vi "LV21_2.vi"() -> ()   [LabVIEW 2021]
panel:
  out "Numeric 3":i32
  out "Real Input 2":string="B Y\nA X\nC Z\nA Z\nB Y\nB Y\nA X\nC Z\nB Y\nB Y\nC Z\nC X\nB Y\nC Z\nB Y\nC Z\nA Z\nA Z\nA X\nB Y\nA X\nC Z\nC Y\nC Z\nC Z\nC Z\nA X\nA X\nB Y\nA Z\nB Z\nB Y\nA X\nA X\nC Z\nB Y\nB Y\nB Z\nA Z\nA X\nC Z\nB Z\nA Z\nC Z\nC Z\nC Z\nC Z\nC Z\nC Z\nB X\nA Z\nA Z\nC Z\nC Z\nC Z\nA Y\nC Z\nB Y\nC Z\nC Z\nC Z\nB Y\nB Z\nA X\nA X\nC Z\nB Y\nB Y\nB Z\nA X\nA X\nC Z\nB Y\nC Z\nA X\nC Z\nA X\nC X\nA Y\nA Y\nB Y\nA Y\nC Z\nB Y\nC Z\nC Z\nA X\nC Z\nA Z\nC Z\nA X\nC Z\nB Y\nB Y\nC Z\nB Z\nC Y\nC Z\nB Y\nC Z\nC Z\nB X\nA X\nC Z\nC Z\nB Y\nC Z\nB Y\nA Z\nB Y\nB Z\nA Z\nC Z\nC Z\nC Z\nA Z\nC Z\nA X\nA X\nA Z\nC Z\nA X\nA Z\nC Z\nA Z\nA Y\nB Y\nA Z\nB X\nA X\nC Z\nC Z\nB Y\nC Y\nB Y\nB Z\nB Y\nB Y\nC Z\nC Z\nC Z\nC Z\nA Y\nC Z\nB Z\nA X\nB Y\nA Y\nC Z\nC Z\nC Z\nC Z\nC Z\nB Y\nC Z\nB Y\nC Z\nB Y\nC Z\nC X\nA Y\nA X\nC Y\nB Y\nA Z\nC Z\nC Z\nB Y\nB Y\nA X\nB Y\nA Y\nA X\nA X\nB Y\nA X\nA X\nB Y\nC Z\nC Z\nB Y\nC Z\nA Z\nC Z\nB Z\nC Z\nA Y\nC Z\nB Z\nC Z\nA Y\nA Y\nC Z\nA X\nB Y\nC Z\nA X\nB Y\nB Y\nA X\nA X\nC Z\nB Y\nC Z\nB Z\nC Z\nA X\nC Z\nB Y\nB Y\nA X\nB Z\nC Z\nB Z\nB Y\nB Y\nA Y\nB Z\nA Z\nC Z\nC Z\nA X\nA X\nA X\nC Z\nB Y\nA X\nA Y\nC Z\nA X\nB Y\nA Y\nA Y\nC Z\nC Z\nC Z\nA Z\nB Z\nC Z\nB Y\nC Z\nC Z\nA Y\nA X\nC Z\nB Y\nC Z\nC Z\nB Y\nB Y\nA Y\nC Z\nB Y\nB Y\nA Z\nC Z\nC Z\nC Z\nC Z\nB Z\nC Z\nB Y\nA X\nC Z\nB Z\nA Z\nA X\nC Z\nA X\nA X\nB Y\nC Z\nC Z\nA X\nC Z\nA Y\nC Z\nC Z\nA X\nB Y\nC Z\nB Z\nB Y\nC Z\nA Z\nC Z\nC Z\nA Y\nA Z\nC Z\nC Z\nB Z\nC Z\nB Y\nC Z\nC Z\nA X\nC Z\nC Z\nB Z\nC Z\nB Z\nA X\nB Y\nC Z\nC Z\nC Z\nC Z\nC Z\nA Z\nA Y\nA X\nA X\nC Z\nB X\nA Z\nA X\nC Z\nB Z\nC Z\nB Y\nA Z\nC Z\nB Y\nC Z\nC Y\nA Y\nC Z\nB Y\nB Y\nC Z\nA X\nC Z\nA X\nC X\nA X\nB X\nA X\nC Z\nC Z\nC Z\nB Y\nB Y\nC Z\nB Z\nC Z\nB Y\nA X\nC X\nC Z\nB Y\nA Z\nA X\nB Y\nB Y\nC Z\nC Z\nC Z\nB Y\nA X\nA X\nB Y\nA X\nA Y\nC Z\nB Y\nA X\nA Y\nB Y\nA X\nA X\nC Z\nC Z\nC Z\nC Z\nC Z\nA X\nA X\nB Z\nA Y\nC Z\nA X\nC Z\nB Y\nC Z\nA Z\nC Z\nC Z\nA Y\nB Z\nC Z\nA X\nB Y\nB Y\nC Z\nA Y\nC Z\nC Z\nC Z\nC Z\nC Z\nB Y\nA X\nA X\nB Y\nC Z\nC Z\nA Z\nC Z\nC Z\nC Z\nA Y\nB Z\nB Y\nB Y\nC Z\nA X\nA Y\nC Z\nA X\nA Y\nA X\nC Z\nA Y\nB Z\nB Y\nB Z\nC Z\nC Z\nC Z\nB Z\nB Z\nC Z\nC Z\nC Z\nC Z\nB Y\nB Z\nA Y\nA Y\nB Z\nB X\nA Z\nA X\nC Z\nA X\nA Y\nA X\nA X\nA X\nC Z\nC Z\nC Z\nA X\nC Z\nC Z\nB Y\nA X\nC Z\nA X\nA Y\nA X\nC Z\nA Y\nC Z\nB Y\nA X\nA Y\nA Z\nC Z\nB Y\nB Y\nB Z\nA X\nA X\nB Y\nC Z\nA X\nB Y\nC Z\nC Z\nC Z\nA X\nA Y\nA Z\nC Z\nB Y\nC Z\nA X\nA Z\nA Z\nB Y\nB Y\nA X\nB Y\nC Z\nB Z\nC Z\nB Y\nA Z\nC Z\nA Y\nA X\nA Z\nB Y\nA X\nA Z\nC Z\nA Z\nC Z\nC Z\nA X\nC Z\nA X\nC Z\nA X\nC Z\nB Y\nC Z\nA X\nB Y\nA Y\nC X\nA Y\nA Z\nA X\nA Z\nB Y\nA X\nC Z\nA Y\nB Y\nB Y\nC Z\nB Y\nC Z\nB Y\nB Z\nC Z\nC Z\nB Y\nA X\nC Z\nB Y\nC Z\nC Z\nC Z\nC Z\nC Z\nA X\nA X\nA Z\nA Z\nC Z\nA Y\nB Y\nA Y\nA Y\nB Y\nC X\nA Y\nC Z\nC Z\nC Z\nA Y\nA Y\nA Y\nC Z\nA X\nB Y\nA X\nB X\nA Y\nA Y\nA X\nB Z\nB Y\nC Z\nB Y\nC Z\nB Y\nC Z\nA Z\nC Z\nA X\nB Y\nA X\nC Z\nB Z\nC Z\nB Y\nC Z\nC Z\nC Z\nA X\nA X\nB Y\nB Z\nA Z\nA X\nA X\nC Z\nA X\nA X\nC X\nC X\nC Z\nB Y\nB Z\nC Z\nA X\nB Y\nB Y\nA Z\nC Z\nC Y\nA X\nB Y\nB Y\nC Y\nA X\nA X\nA X\nA X\nA Z\nB Y\nA Z\nC Z\nC Z\nB Y\nB Z\nB Y\nA Y\nC Z\nC Z\nB Y\nA Y\nC Z\nA X\nC Z\nC Z\nA X\nB Y\nC Z\nC Z\nA X\nA Z\nC Z\nA Z\nC Z\nB Z\nA X\nA Y\nB Y\nA X\nA Y\nA Z\nA Y\nA X\nA Y\nC Z\nA X\nC Z\nC Z\nA X\nA Y\nA X\nC Z\nA Z\nC Z\nC Z\nC Z\nA X\nB Y\nA X\nC Z\nC Z\nC Z\nC Z\nA X\nC Z\nC Z\nB Y\nA Y\nA X\nA X\nC Z\nC Z\nA X\nC Z\nC Z\nB Y\nC Z\nA X\nC Z\nC Z\nA Y\nA X\nC Z\nA Y\nC Z\nA X\nB Z\nB Y\nA X\nB Y\nC Z\nA X\nC Z\nC Z\nA X\nC Z\nB X\nC Z\nC Z\nA Y\nC Z\nA Y\nB X\nC Z\nB Y\nC Z\nA Z\nC Z\nA X\nC Z\nC Z\nC Z\nC Z\nA X\nB X\nC Z\nC Z\nB Y\nA Z\nA Y\nC Z\nA X\nA Z\nA X\nA X\nB Y\nA X\nC Z\nA X\nA X\nB Y\nA X\nB Z\nC Z\nA Z\nA Y\nA X\nB Y\nA X\nA Z\nA X\nB Y\nB Z\nB Y\nC Z\nB Y\nA X\nA Y\nC Z\nA X\nB Z\nC Z\nC Z\nA X\nA X\nA Y\nC Z\nC Z\nC Z\nA Y\nB Y\nA X\nC Z\nB Y\nB Y\nA X\nA X\nB Y\nC Z\nB Y\nA X\nA Z\nC Z\nC Z\nC Z\nC Z\nB Z\nC Z\nA Z\nC Z\nA Y\nB Y\nA Y\nC X\nC Z\nC Z\nA Y\nA X\nB Y\nC Z\nA X\nC Z\nA X\nA Y\nA Y\nB Z\nC Y\nB Y\nC Z\nB Y\nA X\nC Z\nC Z\nC Z\nC Z\nB Y\nA X\nB Y\nA Y\nC Z\nB Y\nA Z\nB Z\nC Z\nC Z\nC Z\nC Z\nA Y\nA X\nC Z\nA X\nC Z\nC Z\nC Z\nC Z\nC Z\nB X\nC Z\nB Z\nA X\nA X\nA Y\nA X\nA Z\nB Y\nA Y\nC Z\nC Z\nC Z\nC Z\nC X\nA Y\nC Z\nC Z\nB Y\nA X\nC Y\nB Y\nC Z\nC Z\nC Z\nB X\nA X\nC Z\nA X\nC Z\nC Z\nC Z\nC Y\nA X\nC Z\nA Z\nC Z\nC Z\nB Y\nA X\nA X\nA Z\nA Y\nC Z\nC Z\nC Z\nC Z\nC Z\nC Z\nC Z\nB Y\nA Y\nA X\nC Z\nC Z\nA X\nA X\nC Z\nC Z\nB Y\nA X\nA X\nC Z\nC Z\nC Z\nB Y\nA Y\nB Z\nA Y\nC Z\nA X\nC Z\nC Z\nB Y\nA Y\nA X\nB Z\nA X\nC Z\nC Z\nC Z\nC Z\nB Z\nC Z\nB Y\nC Z\nC Z\nC Z\nB Y\nC Z\nC Y\nB Z\nB Z\nA Y\nC Z\nC Z\nB Z\nB Y\nC Z\nB Y\nC Z\nC Z\nB Y\nC Z\nC Z\nC Z\nA Y\nA X\nB Y\nC Z\nC Z\nC Z\nB Y\nC Z\nA Y\nA X\nA Z\nA Y\nC Z\nC Z\nC Z\nB Z\nC Z\nB Y\nC Z\nB Y\nA Y\nC Z\nC Z\nA Z\nB Y\nA X\nA X\nB Z\nA X\nC Z\nC Z\nC Z\nA X\nB Z\nC Z\nA X\nC Z\nC Z\nC Z\nC Z\nC Z\nC Z\nA Y\nC Z\nA Z\nA X\nB Y\nC Z\nC Z\nA X\nA Y\nC Z\nB Y\nA X\nC Z\nC Z\nA X\nA Y\nA X\nB Z\nC Z\nA X\nC Z\nA X\nA Z\nB Y\nC Z\nC Z\nC X\nB Z\nB X\nB Y\nA Z\nC Z\nA X\nB Z\nA X\nB Y\nC Z\nB Z\nA Z\nA Z\nC Z\nC Z\nC Z\nC Z\nB Y\nB Y\nA Y\nA X\nA X\nB Y\nA Z\nA X\nC Z\nB Z\nA X\nA X\nB Y\nA X\nC Z\nA X\nC Z\nC Z\nC Z\nC Z\nA X\nA X\nA Z\nC Z\nA X\nB Z\nC Z\nB Y\nC Z\nC Z\nA Y\nC Z\nB Z\nC Z\nC Z\nB Y\nC Z\nC Z\nB Y\nA X\nA X\nC Z\nC Z\nC Z\nA X\nC Z\nC Z\nB Y\nC Z\nB Z\nC Z\nA X\nC Z\nA X\nC Z\nA Y\nC Z\nC Z\nA X\nB Y\nC Z\nC Z\nC Z\nA X\nB Y\nC Z\nA X\nB Z\nA X\nB Z\nC Z\nA X\nC Z\nB Y\nA Z\nB X\nA Y\nC Z\nC Z\nB X\nA Y\nA X\nC Z\nA X\nC Z\nB X\nA X\nB Y\nA Z\nA X\nC Z\nA Y\nC Z\nA X\nC Z\nC Z\nC Z\nC Z\nA Z\nC Z\nC Z\nB Y\nA X\nB Y\nC Z\nB Y\nA X\nC Z\nC Z\nA X\nA X\nB Y\nC Z\nB Y\nC Z\nC Z\nA Z\nC Z\nC Z\nC Z\nA Y\nA Z\nC Z\nC Z\nC Z\nC Z\nA X\nC Z\nA X\nA X\nB Z\nC Z\nC Z\nC Z\nB Z\nA X\nC Z\nA Y\nB Y\nC Z\nA Y\nC Z\nC Z\nA X\nA X\nB Y\nA Z\nA Y\nA X\nB X\nB Y\nB Z\nB Y\nA X\nC Z\nC Z\nB Z\nB Z\nB Z\nC Z\nC Z\nB Y\nB Y\nB Y\nC Z\nB Y\nA X\nA Z\nB Z\nA X\nB Z\nA X\nC Z\nB Y\nB X\nA X\nC Z\nA X\nC Z\nC Z\nC Z\nB X\nB Y\nA Y\nA X\nA X\nA Y\nC Z\nC Z\nB Y\nC Z\nB Z\nA X\nC Z\nC Z\nC Z\nA X\nA Y\nC Z\nB Z\nA X\nA Y\nA Z\nC Z\nB Y\nB Z\nA X\nC Z\nA X\nA X\nA Z\nC Z\nC Z\nB Y\nA X\nC Z\nA Y\nA Z\nA X\nA X\nC Z\nA Y\nB Y\nC Z\nA Z\nC Z\nB Y\nA X\nA X\nA X\nC Y\nC Z\nA Y\nB Z\nC X\nA X\nA X\nA X\nA X\nB Z\nB Y\nC Z\nB Y\nA X\nB Y\nC Z\nB Y\nC Z\nC Z\nA X\nB Y\nA Y\nB X\nA X\nB X\nC Z\nA Z\nA X\nB Y\nB Y\nC Z\nA X\nA X\nB Y\nC Z\nA X\nC Z\nA X\nA Z\nA Z\nC Z\nA Z\nC Z\nC Z\nC Z\nC Z\nA Z\nC Y\nC Z\nC Z\nA Z\nA Y\nA X\nB Z\nC Z\nC Z\nC Z\nA Y\nC Z\nC Z\nC Z\nC Z\nA Z\nB Z\nA X\nC Z\nC Z\nA Y\nB Y\nA X\nC Z\nA X\nB Y\nA X\nA X\nA Z\nB Y\nC Z\nB X\nC X\nA X\nA X\nA X\nC Z\nC Z\nA X\nB Y\nA Z\nB Y\nA X\nA Y\nC Z\nB Y\nC Z\nB Y\nA Y\nB Y\nA Y\nA X\nC Z\nC Z\nA X\nB Y\nA X\nC Z\nC Z\nA Y\nB Y\nB Y\nA Z\nB Y\nC Z\nC Z\nC Z\nB Y\nA X\nB Y\nA X\nC Z\nC Z\nC Z\nA X\nC Z\nC Z\nB Y\nC Z\nB Z\nB Y\nA X\nB Y\nA Z\nB Y\nA X\nB X\nC Z\nA Z\nB Y\nC Z\nB Y\nC Z\nC Z\nC Z\nC Z\nB X\nA X\nB Y\nB Y\nA X\nC Z\nA X\nB Z\nB Z\nB Z\nA X\nC X\nA X\nA X\nA X\nB Y\nB Y\nC Z\nC Z\nA X\nC Z\nB Y\nA X\nC Z\nA X\nC Z\nA X\nB Y\nC Z\nC Z\nA Y\nB Y\nC Z\nA Z\nC Z\nA X\nC Z\nC Z\nA Z\nA Y\nC Z\nA X\nB Y\nB Z\nC Z\nA Y\nA Y\nC Z\nC Z\nB Z\nA Z\nC Z\nA X\nC Z\nA X\nC Z\nC Z\nC Z\nB Y\nC Y\nB Y\nA Y\nA X\nC Z\nB Y\nC Z\nC Z\nC Z\nA Z\nC X\nA Y\nC Z\nA Y\nA Y\nC Z\nA Z\nC Z\nC Z\nC Z\nC Z\nC Z\nB Y\nA Y\nB Y\nA Z\nB Y\nA X\nA X\nB Y\nA Z\nB Y\nC Z\nB Z\nA X\nC Z\nA Y\nA Y\nC Z\nA X\nA X\nC Z\nC Z\nC Z\nB Y\nA X\nC Z\nB Y\nC Z\nB X\nC Z\nA Y\nC Z\nA X\nC Z\nA X\nC Z\nC Z\nB Y\nC Z\nB Z\nC Z\nA Y\nA X\nA Z\nC Z\nC Z\nC Z\nC Z\nC Z\nA Z\nB Y\nB Y\nB Y\nC Z\nC Z\nC X\nC Z\nA X\nB Y\nC Z\nC Z\nA X\nB Y\nC Z\nC Z\nC Z\nC Z\nC Z\nC Z\nA X\nB Z\nC Z\nC Z\nC Z\nA X\nB Z\nC Z\nA X\nC Z\nA Y\nB Y\nC Z\nB Z\nB Y\nC Z\nB X\nC Z\nB Y\nB Y\nB Y\nA X\nA X\nC Z\nA Z\nC Z\nB Y\nB Z\nC Z\nC Z\nB Z\nB Y\nA Z\nB Y\nA X\nA X\nC Z\nC Z\nC Z\nB Y\nA X\nC Z\nC Z\nA Y\nC Z\nB Y\nC Z\nC Z\nC Z\nC Z\nC Z\nC Z\nB Y\nB Y\nC Z\nA Z\nA X\nB Y\nC Z\nB Y\nA X\nA Z\nC Z\nB Y\nA Z\nC Z\nB Y\nA Z\nA X\nB Z\nA X\nC Z\nB Y\nC Z\nA Y\nC Y\nA X\nA Y\nC Z\nC Z\nB Y\nC Z\nB Y\nA Z\nC Z\nC Z\nA X\nC Z\nB Z\nA Y\nB Z\nA Z\nA X\nB Y\nA Z\nA Y\nC Z\nC Z\nB Y\nA X\nB Y\nC Z\nA X\nB Y\nB Y\nC Z\nA Z\nA X\nC Z\nB X\nC Z\nC Z\nC Z\nC Y\nA Z\nA X\nC Z\nC Z\nA X\nB Y\nC Z\nB Y\nC Z\nB Z\nA Z\nC Z\nB Y\nA X\nC Z\nC Z\nB Z\nC Z\nA Z\nB Y\nB Z\nC Z\nC Z\nA X\nC Y\nB Y\nC Z\nA X\nC Z\nC Z\nB Y\nB Z\nC Z\nC Z\nA Y\nA X\nC Z\nA X\nB Z\nB Y\nA Z\nB Z\nC X\nA X\nC Z\nC Z\nC Z\nA X\nB Z\nC Z\nC Z\nC Z\nB Y\nC Z\nA X\nC Z\nC Z\nB Y\nC Z\nA X\nC Z\nC Z\nC Z\nA X\nA X\nB Y\nC Z\nC Z\nB Y\nB Z\nB Y\nC Z\nA X\nA X\nB Y\nA X\nB Y\nC Z\nA X\nC Z\nC Z\nB Z\nA X\nB Y\nC Z\nC Z\nC Z\nC Z\nA Z\nC Z\nA X\nB Y\nA Y\nA Y\nC Z\nC Z\nC Z\nB Y\nA Z\nA X\nB Y\nC Z\nA X\nC Z\nA X\nC Z\nA X\nC Z\nC Z\nB Y\nA Y\nC Z\nB Y\nB Y\nA X\nC Z\nA Y\nA Z\nC Z\nC Z\nC Z\nA Y\nB Y\nC Z\nC Z\nB Z\nC Z\nB Z\nB Y\nA X\nA X\nC Z\nB Z\nC Z\nC Z\nA X\nA X\nB Z\nA X\nC Z\nC Z\nB Y\nA X\nC Z\nA X\nB Y\nC X\nA Z\nB Y\nC Z\nA X\nB Y\nC Z\nA X\nB Y\nC Z\nB X\nC Z\nA Y\nC Z\nA X\nC X\nB Z\nC Z\nB Y\nB Y\nB Y\nA Y\nA X\nC Z\nC Z\nA Y\nB Y\nA X\nC Z\nA X\nC Z\nC Z\nA X\nC Z\nA X\nC Z\nB Y\nC Z\nA X\nA Z\nC X\nB Y\nC Z\nC Z\nB Z\nA X\nA X\nB Y\nC Z\nA Y\nB Y\nC Z\nA X\nA Z\nA X\nB Y\nA X\nB Y\nC Z\nC Z\nB Y\nA X\nB Y\nB Z\nC Z\nB Z\nA X\nC Z\nC Z\nA Y\nC Z\nA X\nC Z\nB Y\nC Z\nC Z\nC Y\nC Z\nC Z\nA Y\nC Z\nC Z\nA Z\nA X\nB Z\nC Z\nA Y\nA X\nB Z\nC Z\nC Z\nB Y\nB Z\nA X\nA X\nC Z\nB Y\nA Y\nC Z\nA Z\nA X\nC Z\nA X\nC Z\nC Z\nA Z\nC Z\nC Z\nC Z\nA Y\nB Y\nA X\nB Z\nB Y\nC Z\nC Z\nC Z\nC Z\nC Z\nC Z\nC Z\nA Z\nB Z\nB X\nA X\nA Z\nA X\nA X\nB Y\nC Z\nC Z\nA X\nB Y\nA Y\nC Z\nB Z\nC Z\nA X\nB Y\nC Z\nB Y\nA Z\nC Z\nA Y\nC Z\nA X\nC Z\nA Z\nB Y\nA Y\nA X\nA X\nA Z\nC Z\nC Z\nC Y\nC Z\nA Y\nA X\nB Y\nA Z\nB Z\nB Z\nC Z\nC Z\nC Z\nC Z\nA X\nA Y\nB Y\nC Z\nB Y\nC Z\nA X\nB Y\nC Z\nC Z\nA Z\nA X\nB Y\nC Z\nA Y\nC Z\nC Z\nC Z\nA X\nB Y\nA X\nB Y\nC Z\nC Z\nB Y\nC Z\nA X\nA X\nC Z\nB Y\nB Z\nA X\nA X\nA X\nC Z\nC Z\nB Y\nA X\nC Z\nA X\nA Z\nC Z\nC Z\nC Z\nC Z\nA Z\nA X\nB X\nB Z\nA Y\nC Z\nC Y\nB Y\nC Z\nA Y\nA X\nB Z\nB Y\nC Z\nB Y\nC Z\nA X\nA Z\nA X\nC Z\nB Y\nB Y\nB Y\nA Z\nC Z\nC Z\nB Y\nC Z\nB Y\nA X\nB Y\nA X\nB Y\nC Z\nC Z\nB Y\nA X\nA Y\nB Z\nC Z\nC Z\nA X\nB Y\nA X\nA X\nA Y\nB X\nA X\nA X\nC Z\nB Z\nA X\nC Z\nA Y\nA Z\nC Z\nA Z\nA X\nB Y\nA X\nC X\nC Z\nB Y\nC Z\nA X\nA X\nC Z\nA X\nB Y\nA X\nC Z\nB Z\nC Z\nA X\nC X\nC Z\nC Z\nA X\nC Z\nA Y\nC Z\nA X\nB Y\nB Y\nB Y\nB Y\nB Y\nB Y\nB Y\nB Y\nA Y\nA Z\nB Y\nC Z\nC Z\nB Y\nA Z\nA X\nA Y\nA X\nC Z\nA Y\nA Z\nA Y\nB Y\nC Z\nC Z\nA Y\nC Z\nA X\nB Y\nC Z\nA X\nC Z\nA X\nB Y\nC Z\nC Z\nA Z\nA X\nC Z\nB Y\nA Z\nC Z\nA X\nC Z\nB Y\nB Y\nC Z\nC Z\nC Z\nC Z\nB Z\nC Z\nC Z\nC Z\nC Z\nC Z\nB Y\nB Y\nA X\nC Z\nC Z\nA Z\nC Z\nA X\nC Z\nC Z\nA X\nB Y\nA X\nC Z\nB Y\nB Y\nA Y\nA Y\nA X\nA Y\nA Y\nC Z\nC Z\nA Y\nC Z\nA Y\nB Y\nC Z\nC Z\nC Z\nB Y\nB Y\nB Y\nA X\nC Z\nB Y\nC Z\nC Z\nC Z\nC Z\nA X\nB Y\nA X\nC Z\nA X\nC Y\nA Y\nB Y\nC Z\nC Z\nC Z\nC Z\nB Y\nC Z\nC Z\nB Y\nC Z\nA X\nA X\nB Y\nB X\nC Z\nB Y\nA X\nB Z\nA Z\nC Z\nC Z\nC Z\nC Z\nB Y\nA Z\nC Z\nC Z\nC Z\nC Z\nA X\nA X\nB Y\nA Z\nC Z\nC Z\nC Z\nC Z\nA Z\nB Y\nA X\nB Y\nC Z\nC Z\nB Z\nC Z\nA Y\nC Z\nA Y\nB Y\nC Z\nA X\nC Z\nA X\nB Z\nB Y\nB Y\nA X\nB X\nA X\nC Z\nB Y\nA X\nA Z\nC Z\nC Z\nA Z\nC Z\nC Z\nB Y\nC Y\nC Z\nA Z\nA Z\nC Z\nB X\nC Z\nC Z\nB Y\nC Z\nB Y\nB Y\nA X\nA Y\nB Y\nA X\nB Z\nC Z\nA Z\nA X\nA X\nA Z\nA Z\nB Z\nA X\nB Y\nC Z\nB Y\nA X\nC Z\nB Z\nA Y\nB Z\nC Z\nA X\nB Z\nA X\nA Y\nC Z\nC Z\nC Z\nC Z\nC Z\nA Y\nA Y\nA X\nB Y\nC Z\nA X\nB Y\nA X\nB Y\nC Z\nA Z\nC Z\nC Z\nC Z\nC Z\nC Z\nB Y\nB Z\nC Z\nA X\nA Z\nA X\nA X\nC Z\nC Z\nC Z\nC Z\nB Y\nC Z\nA X\nC Z\nC Z\nC Z\nC Z\nC Z\nB Y\nA Z\nA X\nA Z\nC Z\nC Z\nC Z\nC Z\nB X\nC Z\nC Z\nA X\nC Z\nA Z\nB Z\nB Y\nB Z\nA Y\nB Y\nB Y\nC Z\nA Y\nA Y\nA Y\nC Z\nC Z\nB Z\nA X\nC Z\nA X\nA X\nA X\nC Z\nC Z\nA Z\nA X\nA Y\nC Z\nC Z\nA X\nB Z\nC Z\nA X\nC Z\nA Z\nA X\nC Z\nC Z\nA X\nA Z\nB Y\nA X\nB Y\nC Z\nC Z\nA X\nB Z\nC Z\nB Y\nC Z\nA Z\nC Z\nA X\nB Y\nC Z\nC Z\nA Y\nC X\nA Y\nA Y\nC Z\nC Z\nA X\nA Z\nB Y\nC Z\nB Y\nC Z\nA Y\nC Z\nC Z\nC Z\nA Z\nC Z\nC Z\nB Y\nA Y\nC Z\nC Z\nB Y\nA X\nC Z\nB Y\nC Z\nB Y\nC Z\nB Y\nA X\nA Y\nB Y\nC Z\nB Z\nA Y\nC Z\nA Y\nA Z\nC Z\nB Y\nC Z\nC Z\nB Y\nA Y\nA Y\nC Z\nC Z\nA Y\nC Z\nC X\nC Z\nC Z\nC Z\nA X\nC Z\nB Y\nB Y\nC Z\nC Y\nB Z\nC Z\nB Y\nA X\nA X\nB Y\nC Z\nA X\nC Z\nB Z\nC Z\nA X\nB Y"
  out "Real Input":string
  out "Numeric":i32
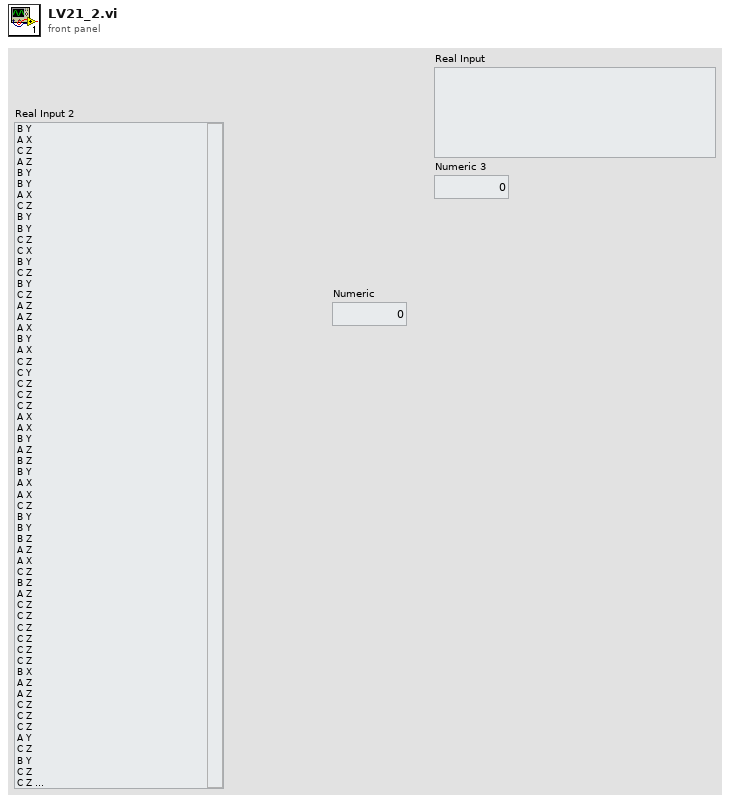
[diagram p1: front panel]
types:
  T1 = enum16{"NOT DEFINED", "Rock", "Paper", "Scissors"}
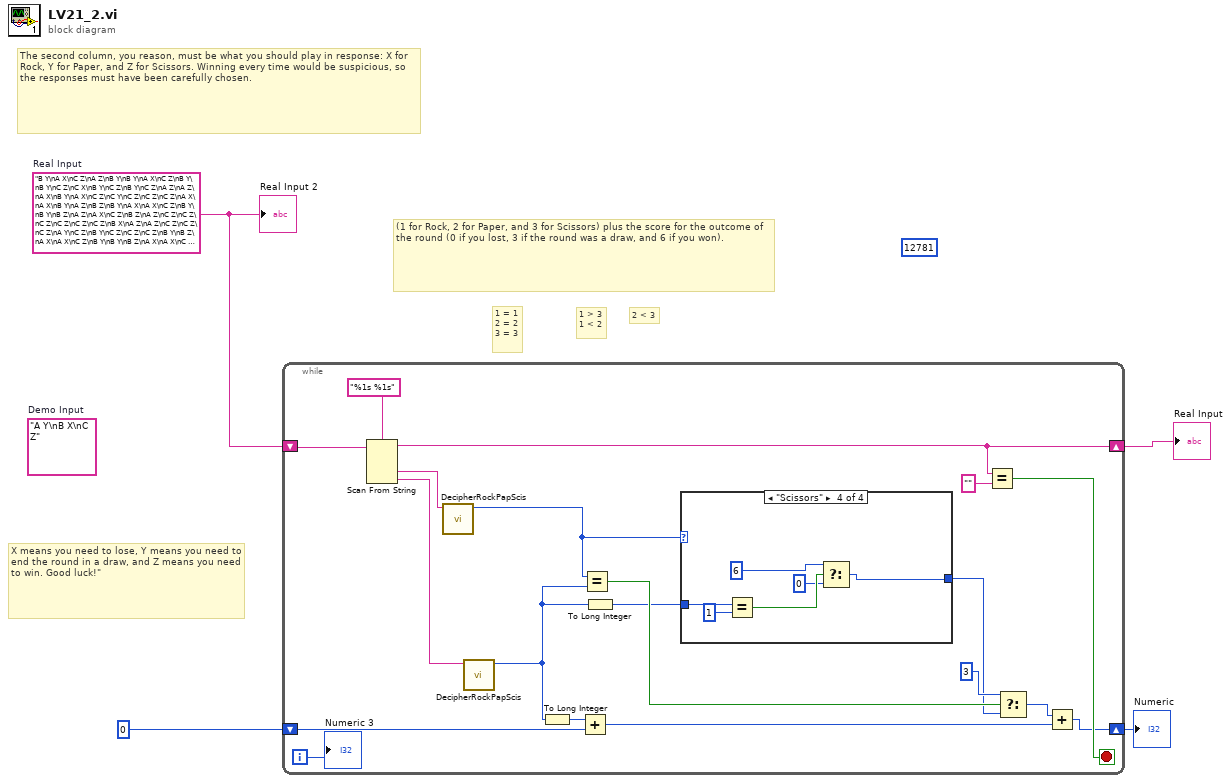
[diagram p0: block diagram]
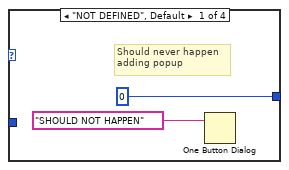
[diagram p2: hidden frame]
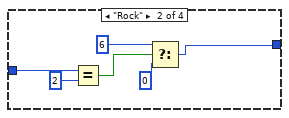
[diagram p3: hidden frame]
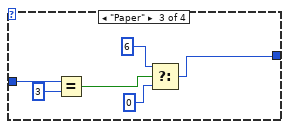
[diagram p4: hidden frame]
diagram:
  (unwired) 12781 ("Numeric 2")
  (unwired) "A Y\nB X\nC Z"  # Demo Input
  w1 = "B Y\nA X\nC Z\nA Z\nB Y\nB Y\nA X\nC Z\nB Y\nB Y\nC Z\nC X\nB Y\nC Z\nB Y\nC Z\nA Z\nA Z\nA X\nB Y\nA X\nC Z\nC Y\nC Z\nC Z\nC Z\nA X\nA X\nB Y\nA Z\nB Z\nB Y\nA X\nA X\nC Z\nB Y\nB Y\nB Z\nA Z\nA X\nC Z\nB Z\nA Z\nC Z\nC Z\nC Z\nC Z\nC Z\nC Z\nB X\nA Z\nA Z\nC Z\nC Z\nC Z\nA Y\nC Z\nB Y\nC Z\nC Z\nC Z\nB Y\nB Z\nA X\nA X\nC Z\nB Y\nB Y\nB Z\nA X\nA X\nC Z\nB Y\nC Z\nA X\nC Z\nA X\nC X\nA Y\nA Y\nB Y\nA Y\nC Z\nB Y\nC Z\nC Z\nA X\nC Z\nA Z\nC Z\nA X\nC Z\nB Y\nB Y\nC Z\nB Z\nC Y\nC Z\nB Y\nC Z\nC Z\nB X\nA X\nC Z\nC Z\nB Y\nC Z\nB Y\nA Z\nB Y\nB Z\nA Z\nC Z\nC Z\nC Z\nA Z\nC Z\nA X\nA X\nA Z\nC Z\nA X\nA Z\nC Z\nA Z\nA Y\nB Y\nA Z\nB X\nA X\nC Z\nC Z\nB Y\nC Y\nB Y\nB Z\nB Y\nB Y\nC Z\nC Z\nC Z\nC Z\nA Y\nC Z\nB Z\nA X\nB Y\nA Y\nC Z\nC Z\nC Z\nC Z\nC Z\nB Y\nC Z\nB Y\nC Z\nB Y\nC Z\nC X\nA Y\nA X\nC Y\nB Y\nA Z\nC Z\nC Z\nB Y\nB Y\nA X\nB Y\nA Y\nA X\nA X\nB Y\nA X\nA X\nB Y\nC Z\nC Z\nB Y\nC Z\nA Z\nC Z\nB Z\nC Z\nA Y\nC Z\nB Z\nC Z\nA Y\nA Y\nC Z\nA X\nB Y\nC Z\nA X\nB Y\nB Y\nA X\nA X\nC Z\nB Y\nC Z\nB Z\nC Z\nA X\nC Z\nB Y\nB Y\nA X\nB Z\nC Z\nB Z\nB Y\nB Y\nA Y\nB Z\nA Z\nC Z\nC Z\nA X\nA X\nA X\nC Z\nB Y\nA X\nA Y\nC Z\nA X\nB Y\nA Y\nA Y\nC Z\nC Z\nC Z\nA Z\nB Z\nC Z\nB Y\nC Z\nC Z\nA Y\nA X\nC Z\nB Y\nC Z\nC Z\nB Y\nB Y\nA Y\nC Z\nB Y\nB Y\nA Z\nC Z\nC Z\nC Z\nC Z\nB Z\nC Z\nB Y\nA X\nC Z\nB Z\nA Z\nA X\nC Z\nA X\nA X\nB Y\nC Z\nC Z\nA X\nC Z\nA Y\nC Z\nC Z\nA X\nB Y\nC Z\nB Z\nB Y\nC Z\nA Z\nC Z\nC Z\nA Y\nA Z\nC Z\nC Z\nB Z\nC Z\nB Y\nC Z\nC Z\nA X\nC Z\nC Z\nB Z\nC Z\nB Z\nA X\nB Y\nC Z\nC Z\nC Z\nC Z\nC Z\nA Z\nA Y\nA X\nA X\nC Z\nB X\nA Z\nA X\nC Z\nB Z\nC Z\nB Y\nA Z\nC Z\nB Y\nC Z\nC Y\nA Y\nC Z\nB Y\nB Y\nC Z\nA X\nC Z\nA X\nC X\nA X\nB X\nA X\nC Z\nC Z\nC Z\nB Y\nB Y\nC Z\nB Z\nC Z\nB Y\nA X\nC X\nC Z\nB Y\nA Z\nA X\nB Y\nB Y\nC Z\nC Z\nC Z\nB Y\nA X\nA X\nB Y\nA X\nA Y\nC Z\nB Y\nA X\nA Y\nB Y\nA X\nA X\nC Z\nC Z\nC Z\nC Z\nC Z\nA X\nA X\nB Z\nA Y\nC Z\nA X\nC Z\nB Y\nC Z\nA Z\nC Z\nC Z\nA Y\nB Z\nC Z\nA X\nB Y\nB Y\nC Z\nA Y\nC Z\nC Z\nC Z\nC Z\nC Z\nB Y\nA X\nA X\nB Y\nC Z\nC Z\nA Z\nC Z\nC Z\nC Z\nA Y\nB Z\nB Y\nB Y\nC Z\nA X\nA Y\nC Z\nA X\nA Y\nA X\nC Z\nA Y\nB Z\nB Y\nB Z\nC Z\nC Z\nC Z\nB Z\nB Z\nC Z\nC Z\nC Z\nC Z\nB Y\nB Z\nA Y\nA Y\nB Z\nB X\nA Z\nA X\nC Z\nA X\nA Y\nA X\nA X\nA X\nC Z\nC Z\nC Z\nA X\nC Z\nC Z\nB Y\nA X\nC Z\nA X\nA Y\nA X\nC Z\nA Y\nC Z\nB Y\nA X\nA Y\nA Z\nC Z\nB Y\nB Y\nB Z\nA X\nA X\nB Y\nC Z\nA X\nB Y\nC Z\nC Z\nC Z\nA X\nA Y\nA Z\nC Z\nB Y\nC Z\nA X\nA Z\nA Z\nB Y\nB Y\nA X\nB Y\nC Z\nB Z\nC Z\nB Y\nA Z\nC Z\nA Y\nA X\nA Z\nB Y\nA X\nA Z\nC Z\nA Z\nC Z\nC Z\nA X\nC Z\nA X\nC Z\nA X\nC Z\nB Y\nC Z\nA X\nB Y\nA Y\nC X\nA Y\nA Z\nA X\nA Z\nB Y\nA X\nC Z\nA Y\nB Y\nB Y\nC Z\nB Y\nC Z\nB Y\nB Z\nC Z\nC Z\nB Y\nA X\nC Z\nB Y\nC Z\nC Z\nC Z\nC Z\nC Z\nA X\nA X\nA Z\nA Z\nC Z\nA Y\nB Y\nA Y\nA Y\nB Y\nC X\nA Y\nC Z\nC Z\nC Z\nA Y\nA Y\nA Y\nC Z\nA X\nB Y\nA X\nB X\nA Y\nA Y\nA X\nB Z\nB Y\nC Z\nB Y\nC Z\nB Y\nC Z\nA Z\nC Z\nA X\nB Y\nA X\nC Z\nB Z\nC Z\nB Y\nC Z\nC Z\nC Z\nA X\nA X\nB Y\nB Z\nA Z\nA X\nA X\nC Z\nA X\nA X\nC X\nC X\nC Z\nB Y\nB Z\nC Z\nA X\nB Y\nB Y\nA Z\nC Z\nC Y\nA X\nB Y\nB Y\nC Y\nA X\nA X\nA X\nA X\nA Z\nB Y\nA Z\nC Z\nC Z\nB Y\nB Z\nB Y\nA Y\nC Z\nC Z\nB Y\nA Y\nC Z\nA X\nC Z\nC Z\nA X\nB Y\nC Z\nC Z\nA X\nA Z\nC Z\nA Z\nC Z\nB Z\nA X\nA Y\nB Y\nA X\nA Y\nA Z\nA Y\nA X\nA Y\nC Z\nA X\nC Z\nC Z\nA X\nA Y\nA X\nC Z\nA Z\nC Z\nC Z\nC Z\nA X\nB Y\nA X\nC Z\nC Z\nC Z\nC Z\nA X\nC Z\nC Z\nB Y\nA Y\nA X\nA X\nC Z\nC Z\nA X\nC Z\nC Z\nB Y\nC Z\nA X\nC Z\nC Z\nA Y\nA X\nC Z\nA Y\nC Z\nA X\nB Z\nB Y\nA X\nB Y\nC Z\nA X\nC Z\nC Z\nA X\nC Z\nB X\nC Z\nC Z\nA Y\nC Z\nA Y\nB X\nC Z\nB Y\nC Z\nA Z\nC Z\nA X\nC Z\nC Z\nC Z\nC Z\nA X\nB X\nC Z\nC Z\nB Y\nA Z\nA Y\nC Z\nA X\nA Z\nA X\nA X\nB Y\nA X\nC Z\nA X\nA X\nB Y\nA X\nB Z\nC Z\nA Z\nA Y\nA X\nB Y\nA X\nA Z\nA X\nB Y\nB Z\nB Y\nC Z\nB Y\nA X\nA Y\nC Z\nA X\nB Z\nC Z\nC Z\nA X\nA X\nA Y\nC Z\nC Z\nC Z\nA Y\nB Y\nA X\nC Z\nB Y\nB Y\nA X\nA X\nB Y\nC Z\nB Y\nA X\nA Z\nC Z\nC Z\nC Z\nC Z\nB Z\nC Z\nA Z\nC Z\nA Y\nB Y\nA Y\nC X\nC Z\nC Z\nA Y\nA X\nB Y\nC Z\nA X\nC Z\nA X\nA Y\nA Y\nB Z\nC Y\nB Y\nC Z\nB Y\nA X\nC Z\nC Z\nC Z\nC Z\nB Y\nA X\nB Y\nA Y\nC Z\nB Y\nA Z\nB Z\nC Z\nC Z\nC Z\nC Z\nA Y\nA X\nC Z\nA X\nC Z\nC Z\nC Z\nC Z\nC Z\nB X\nC Z\nB Z\nA X\nA X\nA Y\nA X\nA Z\nB Y\nA Y\nC Z\nC Z\nC Z\nC Z\nC X\nA Y\nC Z\nC Z\nB Y\nA X\nC Y\nB Y\nC Z\nC Z\nC Z\nB X\nA X\nC Z\nA X\nC Z\nC Z\nC Z\nC Y\nA X\nC Z\nA Z\nC Z\nC Z\nB Y\nA X\nA X\nA Z\nA Y\nC Z\nC Z\nC Z\nC Z\nC Z\nC Z\nC Z\nB Y\nA Y\nA X\nC Z\nC Z\nA X\nA X\nC Z\nC Z\nB Y\nA X\nA X\nC Z\nC Z\nC Z\nB Y\nA Y\nB Z\nA Y\nC Z\nA X\nC Z\nC Z\nB Y\nA Y\nA X\nB Z\nA X\nC Z\nC Z\nC Z\nC Z\nB Z\nC Z\nB Y\nC Z\nC Z\nC Z\nB Y\nC Z\nC Y\nB Z\nB Z\nA Y\nC Z\nC Z\nB Z\nB Y\nC Z\nB Y\nC Z\nC Z\nB Y\nC Z\nC Z\nC Z\nA Y\nA X\nB Y\nC Z\nC Z\nC Z\nB Y\nC Z\nA Y\nA X\nA Z\nA Y\nC Z\nC Z\nC Z\nB Z\nC Z\nB Y\nC Z\nB Y\nA Y\nC Z\nC Z\nA Z\nB Y\nA X\nA X\nB Z\nA X\nC Z\nC Z\nC Z\nA X\nB Z\nC Z\nA X\nC Z\nC Z\nC Z\nC Z\nC Z\nC Z\nA Y\nC Z\nA Z\nA X\nB Y\nC Z\nC Z\nA X\nA Y\nC Z\nB Y\nA X\nC Z\nC Z\nA X\nA Y\nA X\nB Z\nC Z\nA X\nC Z\nA X\nA Z\nB Y\nC Z\nC Z\nC X\nB Z\nB X\nB Y\nA Z\nC Z\nA X\nB Z\nA X\nB Y\nC Z\nB Z\nA Z\nA Z\nC Z\nC Z\nC Z\nC Z\nB Y\nB Y\nA Y\nA X\nA X\nB Y\nA Z\nA X\nC Z\nB Z\nA X\nA X\nB Y\nA X\nC Z\nA X\nC Z\nC Z\nC Z\nC Z\nA X\nA X\nA Z\nC Z\nA X\nB Z\nC Z\nB Y\nC Z\nC Z\nA Y\nC Z\nB Z\nC Z\nC Z\nB Y\nC Z\nC Z\nB Y\nA X\nA X\nC Z\nC Z\nC Z\nA X\nC Z\nC Z\nB Y\nC Z\nB Z\nC Z\nA X\nC Z\nA X\nC Z\nA Y\nC Z\nC Z\nA X\nB Y\nC Z\nC Z\nC Z\nA X\nB Y\nC Z\nA X\nB Z\nA X\nB Z\nC Z\nA X\nC Z\nB Y\nA Z\nB X\nA Y\nC Z\nC Z\nB X\nA Y\nA X\nC Z\nA X\nC Z\nB X\nA X\nB Y\nA Z\nA X\nC Z\nA Y\nC Z\nA X\nC Z\nC Z\nC Z\nC Z\nA Z\nC Z\nC Z\nB Y\nA X\nB Y\nC Z\nB Y\nA X\nC Z\nC Z\nA X\nA X\nB Y\nC Z\nB Y\nC Z\nC Z\nA Z\nC Z\nC Z\nC Z\nA Y\nA Z\nC Z\nC Z\nC Z\nC Z\nA X\nC Z\nA X\nA X\nB Z\nC Z\nC Z\nC Z\nB Z\nA X\nC Z\nA Y\nB Y\nC Z\nA Y\nC Z\nC Z\nA X\nA X\nB Y\nA Z\nA Y\nA X\nB X\nB Y\nB Z\nB Y\nA X\nC Z\nC Z\nB Z\nB Z\nB Z\nC Z\nC Z\nB Y\nB Y\nB Y\nC Z\nB Y\nA X\nA Z\nB Z\nA X\nB Z\nA X\nC Z\nB Y\nB X\nA X\nC Z\nA X\nC Z\nC Z\nC Z\nB X\nB Y\nA Y\nA X\nA X\nA Y\nC Z\nC Z\nB Y\nC Z\nB Z\nA X\nC Z\nC Z\nC Z\nA X\nA Y\nC Z\nB Z\nA X\nA Y\nA Z\nC Z\nB Y\nB Z\nA X\nC Z\nA X\nA X\nA Z\nC Z\nC Z\nB Y\nA X\nC Z\nA Y\nA Z\nA X\nA X\nC Z\nA Y\nB Y\nC Z\nA Z\nC Z\nB Y\nA X\nA X\nA X\nC Y\nC Z\nA Y\nB Z\nC X\nA X\nA X\nA X\nA X\nB Z\nB Y\nC Z\nB Y\nA X\nB Y\nC Z\nB Y\nC Z\nC Z\nA X\nB Y\nA Y\nB X\nA X\nB X\nC Z\nA Z\nA X\nB Y\nB Y\nC Z\nA X\nA X\nB Y\nC Z\nA X\nC Z\nA X\nA Z\nA Z\nC Z\nA Z\nC Z\nC Z\nC Z\nC Z\nA Z\nC Y\nC Z\nC Z\nA Z\nA Y\nA X\nB Z\nC Z\nC Z\nC Z\nA Y\nC Z\nC Z\nC Z\nC Z\nA Z\nB Z\nA X\nC Z\nC Z\nA Y\nB Y\nA X\nC Z\nA X\nB Y\nA X\nA X\nA Z\nB Y\nC Z\nB X\nC X\nA X\nA X\nA X\nC Z\nC Z\nA X\nB Y\nA Z\nB Y\nA X\nA Y\nC Z\nB Y\nC Z\nB Y\nA Y\nB Y\nA Y\nA X\nC Z\nC Z\nA X\nB Y\nA X\nC Z\nC Z\nA Y\nB Y\nB Y\nA Z\nB Y\nC Z\nC Z\nC Z\nB Y\nA X\nB Y\nA X\nC Z\nC Z\nC Z\nA X\nC Z\nC Z\nB Y\nC Z\nB Z\nB Y\nA X\nB Y\nA Z\nB Y\nA X\nB X\nC Z\nA Z\nB Y\nC Z\nB Y\nC Z\nC Z\nC Z\nC Z\nB X\nA X\nB Y\nB Y\nA X\nC Z\nA X\nB Z\nB Z\nB Z\nA X\nC X\nA X\nA X\nA X\nB Y\nB Y\nC Z\nC Z\nA X\nC Z\nB Y\nA X\nC Z\nA X\nC Z\nA X\nB Y\nC Z\nC Z\nA Y\nB Y\nC Z\nA Z\nC Z\nA X\nC Z\nC Z\nA Z\nA Y\nC Z\nA X\nB Y\nB Z\nC Z\nA Y\nA Y\nC Z\nC Z\nB Z\nA Z\nC Z\nA X\nC Z\nA X\nC Z\nC Z\nC Z\nB Y\nC Y\nB Y\nA Y\nA X\nC Z\nB Y\nC Z\nC Z\nC Z\nA Z\nC X\nA Y\nC Z\nA Y\nA Y\nC Z\nA Z\nC Z\nC Z\nC Z\nC Z\nC Z\nB Y\nA Y\nB Y\nA Z\nB Y\nA X\nA X\nB Y\nA Z\nB Y\nC Z\nB Z\nA X\nC Z\nA Y\nA Y\nC Z\nA X\nA X\nC Z\nC Z\nC Z\nB Y\nA X\nC Z\nB Y\nC Z\nB X\nC Z\nA Y\nC Z\nA X\nC Z\nA X\nC Z\nC Z\nB Y\nC Z\nB Z\nC Z\nA Y\nA X\nA Z\nC Z\nC Z\nC Z\nC Z\nC Z\nA Z\nB Y\nB Y\nB Y\nC Z\nC Z\nC X\nC Z\nA X\nB Y\nC Z\nC Z\nA X\nB Y\nC Z\nC Z\nC Z\nC Z\nC Z\nC Z\nA X\nB Z\nC Z\nC Z\nC Z\nA X\nB Z\nC Z\nA X\nC Z\nA Y\nB Y\nC Z\nB Z\nB Y\nC Z\nB X\nC Z\nB Y\nB Y\nB Y\nA X\nA X\nC Z\nA Z\nC Z\nB Y\nB Z\nC Z\nC Z\nB Z\nB Y\nA Z\nB Y\nA X\nA X\nC Z\nC Z\nC Z\nB Y\nA X\nC Z\nC Z\nA Y\nC Z\nB Y\nC Z\nC Z\nC Z\nC Z\nC Z\nC Z\nB Y\nB Y\nC Z\nA Z\nA X\nB Y\nC Z\nB Y\nA X\nA Z\nC Z\nB Y\nA Z\nC Z\nB Y\nA Z\nA X\nB Z\nA X\nC Z\nB Y\nC Z\nA Y\nC Y\nA X\nA Y\nC Z\nC Z\nB Y\nC Z\nB Y\nA Z\nC Z\nC Z\nA X\nC Z\nB Z\nA Y\nB Z\nA Z\nA X\nB Y\nA Z\nA Y\nC Z\nC Z\nB Y\nA X\nB Y\nC Z\nA X\nB Y\nB Y\nC Z\nA Z\nA X\nC Z\nB X\nC Z\nC Z\nC Z\nC Y\nA Z\nA X\nC Z\nC Z\nA X\nB Y\nC Z\nB Y\nC Z\nB Z\nA Z\nC Z\nB Y\nA X\nC Z\nC Z\nB Z\nC Z\nA Z\nB Y\nB Z\nC Z\nC Z\nA X\nC Y\nB Y\nC Z\nA X\nC Z\nC Z\nB Y\nB Z\nC Z\nC Z\nA Y\nA X\nC Z\nA X\nB Z\nB Y\nA Z\nB Z\nC X\nA X\nC Z\nC Z\nC Z\nA X\nB Z\nC Z\nC Z\nC Z\nB Y\nC Z\nA X\nC Z\nC Z\nB Y\nC Z\nA X\nC Z\nC Z\nC Z\nA X\nA X\nB Y\nC Z\nC Z\nB Y\nB Z\nB Y\nC Z\nA X\nA X\nB Y\nA X\nB Y\nC Z\nA X\nC Z\nC Z\nB Z\nA X\nB Y\nC Z\nC Z\nC Z\nC Z\nA Z\nC Z\nA X\nB Y\nA Y\nA Y\nC Z\nC Z\nC Z\nB Y\nA Z\nA X\nB Y\nC Z\nA X\nC Z\nA X\nC Z\nA X\nC Z\nC Z\nB Y\nA Y\nC Z\nB Y\nB Y\nA X\nC Z\nA Y\nA Z\nC Z\nC Z\nC Z\nA Y\nB Y\nC Z\nC Z\nB Z\nC Z\nB Z\nB Y\nA X\nA X\nC Z\nB Z\nC Z\nC Z\nA X\nA X\nB Z\nA X\nC Z\nC Z\nB Y\nA X\nC Z\nA X\nB Y\nC X\nA Z\nB Y\nC Z\nA X\nB Y\nC Z\nA X\nB Y\nC Z\nB X\nC Z\nA Y\nC Z\nA X\nC X\nB Z\nC Z\nB Y\nB Y\nB Y\nA Y\nA X\nC Z\nC Z\nA Y\nB Y\nA X\nC Z\nA X\nC Z\nC Z\nA X\nC Z\nA X\nC Z\nB Y\nC Z\nA X\nA Z\nC X\nB Y\nC Z\nC Z\nB Z\nA X\nA X\nB Y\nC Z\nA Y\nB Y\nC Z\nA X\nA Z\nA X\nB Y\nA X\nB Y\nC Z\nC Z\nB Y\nA X\nB Y\nB Z\nC Z\nB Z\nA X\nC Z\nC Z\nA Y\nC Z\nA X\nC Z\nB Y\nC Z\nC Z\nC Y\nC Z\nC Z\nA Y\nC Z\nC Z\nA Z\nA X\nB Z\nC Z\nA Y\nA X\nB Z\nC Z\nC Z\nB Y\nB Z\nA X\nA X\nC Z\nB Y\nA Y\nC Z\nA Z\nA X\nC Z\nA X\nC Z\nC Z\nA Z\nC Z\nC Z\nC Z\nA Y\nB Y\nA X\nB Z\nB Y\nC Z\nC Z\nC Z\nC Z\nC Z\nC Z\nC Z\nA Z\nB Z\nB X\nA X\nA Z\nA X\nA X\nB Y\nC Z\nC Z\nA X\nB Y\nA Y\nC Z\nB Z\nC Z\nA X\nB Y\nC Z\nB Y\nA Z\nC Z\nA Y\nC Z\nA X\nC Z\nA Z\nB Y\nA Y\nA X\nA X\nA Z\nC Z\nC Z\nC Y\nC Z\nA Y\nA X\nB Y\nA Z\nB Z\nB Z\nC Z\nC Z\nC Z\nC Z\nA X\nA Y\nB Y\nC Z\nB Y\nC Z\nA X\nB Y\nC Z\nC Z\nA Z\nA X\nB Y\nC Z\nA Y\nC Z\nC Z\nC Z\nA X\nB Y\nA X\nB Y\nC Z\nC Z\nB Y\nC Z\nA X\nA X\nC Z\nB Y\nB Z\nA X\nA X\nA X\nC Z\nC Z\nB Y\nA X\nC Z\nA X\nA Z\nC Z\nC Z\nC Z\nC Z\nA Z\nA X\nB X\nB Z\nA Y\nC Z\nC Y\nB Y\nC Z\nA Y\nA X\nB Z\nB Y\nC Z\nB Y\nC Z\nA X\nA Z\nA X\nC Z\nB Y\nB Y\nB Y\nA Z\nC Z\nC Z\nB Y\nC Z\nB Y\nA X\nB Y\nA X\nB Y\nC Z\nC Z\nB Y\nA X\nA Y\nB Z\nC Z\nC Z\nA X\nB Y\nA X\nA X\nA Y\nB X\nA X\nA X\nC Z\nB Z\nA X\nC Z\nA Y\nA Z\nC Z\nA Z\nA X\nB Y\nA X\nC X\nC Z\nB Y\nC Z\nA X\nA X\nC Z\nA X\nB Y\nA X\nC Z\nB Z\nC Z\nA X\nC X\nC Z\nC Z\nA X\nC Z\nA Y\nC Z\nA X\nB Y\nB Y\nB Y\nB Y\nB Y\nB Y\nB Y\nB Y\nA Y\nA Z\nB Y\nC Z\nC Z\nB Y\nA Z\nA X\nA Y\nA X\nC Z\nA Y\nA Z\nA Y\nB Y\nC Z\nC Z\nA Y\nC Z\nA X\nB Y\nC Z\nA X\nC Z\nA X\nB Y\nC Z\nC Z\nA Z\nA X\nC Z\nB Y\nA Z\nC Z\nA X\nC Z\nB Y\nB Y\nC Z\nC Z\nC Z\nC Z\nB Z\nC Z\nC Z\nC Z\nC Z\nC Z\nB Y\nB Y\nA X\nC Z\nC Z\nA Z\nC Z\nA X\nC Z\nC Z\nA X\nB Y\nA X\nC Z\nB Y\nB Y\nA Y\nA Y\nA X\nA Y\nA Y\nC Z\nC Z\nA Y\nC Z\nA Y\nB Y\nC Z\nC Z\nC Z\nB Y\nB Y\nB Y\nA X\nC Z\nB Y\nC Z\nC Z\nC Z\nC Z\nA X\nB Y\nA X\nC Z\nA X\nC Y\nA Y\nB Y\nC Z\nC Z\nC Z\nC Z\nB Y\nC Z\nC Z\nB Y\nC Z\nA X\nA X\nB Y\nB X\nC Z\nB Y\nA X\nB Z\nA Z\nC Z\nC Z\nC Z\nC Z\nB Y\nA Z\nC Z\nC Z\nC Z\nC Z\nA X\nA X\nB Y\nA Z\nC Z\nC Z\nC Z\nC Z\nA Z\nB Y\nA X\nB Y\nC Z\nC Z\nB Z\nC Z\nA Y\nC Z\nA Y\nB Y\nC Z\nA X\nC Z\nA X\nB Z\nB Y\nB Y\nA X\nB X\nA X\nC Z\nB Y\nA X\nA Z\nC Z\nC Z\nA Z\nC Z\nC Z\nB Y\nC Y\nC Z\nA Z\nA Z\nC Z\nB X\nC Z\nC Z\nB Y\nC Z\nB Y\nB Y\nA X\nA Y\nB Y\nA X\nB Z\nC Z\nA Z\nA X\nA X\nA Z\nA Z\nB Z\nA X\nB Y\nC Z\nB Y\nA X\nC Z\nB Z\nA Y\nB Z\nC Z\nA X\nB Z\nA X\nA Y\nC Z\nC Z\nC Z\nC Z\nC Z\nA Y\nA Y\nA X\nB Y\nC Z\nA X\nB Y\nA X\nB Y\nC Z\nA Z\nC Z\nC Z\nC Z\nC Z\nC Z\nB Y\nB Z\nC Z\nA X\nA Z\nA X\nA X\nC Z\nC Z\nC Z\nC Z\nB Y\nC Z\nA X\nC Z\nC Z\nC Z\nC Z\nC Z\nB Y\nA Z\nA X\nA Z\nC Z\nC Z\nC Z\nC Z\nB X\nC Z\nC Z\nA X\nC Z\nA Z\nB Z\nB Y\nB Z\nA Y\nB Y\nB Y\nC Z\nA Y\nA Y\nA Y\nC Z\nC Z\nB Z\nA X\nC Z\nA X\nA X\nA X\nC Z\nC Z\nA Z\nA X\nA Y\nC Z\nC Z\nA X\nB Z\nC Z\nA X\nC Z\nA Z\nA X\nC Z\nC Z\nA X\nA Z\nB Y\nA X\nB Y\nC Z\nC Z\nA X\nB Z\nC Z\nB Y\nC Z\nA Z\nC Z\nA X\nB Y\nC Z\nC Z\nA Y\nC X\nA Y\nA Y\nC Z\nC Z\nA X\nA Z\nB Y\nC Z\nB Y\nC Z\nA Y\nC Z\nC Z\nC Z\nA Z\nC Z\nC Z\nB Y\nA Y\nC Z\nC Z\nB Y\nA X\nC Z\nB Y\nC Z\nB Y\nC Z\nB Y\nA X\nA Y\nB Y\nC Z\nB Z\nA Y\nC Z\nA Y\nA Z\nC Z\nB Y\nC Z\nC Z\nB Y\nA Y\nA Y\nC Z\nC Z\nA Y\nC Z\nC X\nC Z\nC Z\nC Z\nA X\nC Z\nB Y\nB Y\nC Z\nC Y\nB Z\nC Z\nB Y\nA X\nA X\nB Y\nC Z\nA X\nC Z\nB Z\nC Z\nA X\nB Y"  # Real Input
  # "X means you need to lose, Y means you need to end the round in a draw, and Z means you need to win. Good luck!\""
  # "2 < 3"
  # "1 > 3\n1 < 2"
  # "1 = 1\n2 = 2\n3 = 3"
  # "(1 for Rock, 2 for Paper, and 3 for Scissors) plus the score for the outcome of the round (0 if you lost, 3 if the round was a draw, and 6 if you won)."
  # "The second column, you reason, must be what you should play in response: X for Rock, Y for Paper, and Z for Scissors. Winning every time would be suspicious, so the responses must have been carefully chosen."
  n1 = while {
    shift-right: [w21] -> w2
    shift-left: w1 -> [w23]
    shift-right: [w13] -> w3
    shift-left: 0 -> [w15]
    i -> [w5]
    stop <- w19 stop-if-true
    n2 = Scan From String(format string="%1s %1s", input string=w23) -> (remaining string=w21:string, output 1=w18:string, output 2=w17:string)  [unwired: 4 in, 2 out]
    n3 = call "DecipherRockPapScis.vi"("A"=w18) -> ("Enum"=w8:T1)  [unwired: 10 in]
    n4 = call "DecipherRockPapScis.vi"("A"=w17) -> ("Enum"=w9:T1)  [unwired: 10 in]
    n5 = To Long Integer(number=w9) -> (32bit integer=w14:i32)
    n6 = Add(x=w14, y=w15) -> (x+y=w16:i32)
    n7 = Equal?(x=w8, y=w9) -> (x = y?=w10:bool)
    n8 = To Long Integer(number=w9) -> (32bit integer=w7:i32)
    n9 = case shown="\"Scissors\"" w8 {
      tunnel: w7 -> [_ w31 w37 w43]
      tunnel: [0 ("y") w26 w32 w38] -> w6
      frame "NOT DEFINED", Default {
        # "Should never happen\nadding popup"
        n10 = One Button Dialog(message="SHOULD NOT HAPPEN") -> ()  [unwired: 1 in, 1 out]
      }
      frame "Rock" {
        n11 = Equal?(x=w31, y=2) -> (x = y?=w29:bool)
        n12 = Select(t=6 ("y"), s=w29, f=0) -> (s? t:f=w26:i32)
      }
      frame "Paper" {
        n13 = Equal?(x=w37, y=3) -> (x = y?=w35:bool)
        n14 = Select(t=6 ("y"), s=w35, f=0) -> (s? t:f=w32:i32)
      }
      frame "Scissors" {
        n15 = Equal?(x=w43, y=1) -> (x = y?=w40:bool)
        n16 = Select(t=6 ("y"), s=w40, f=0) -> (s? t:f=w38:i32)
      }
    }
    n17 = Equal?(x=w21, y="") -> (x = y?=w19:bool)
    n18 = Select(t=3, s=w10, f=w6) -> (s? t:f=w11:i32)
    n19 = Add(x=w11, y=w16) -> (x+y=w13:i32)
    "Numeric 3" <- w5
  }
  "Numeric" <- w3
  "Real Input" <- w2
  "Real Input 2" <- w1
